vi "DHE_Interlocks.vi"(8 "remaining":string, 9 "field":string, 10 "parent":string, 11 "DHE_ImgState":T1(ring)) -> (2 "interlock closed":bool)   [LabVIEW 2016]
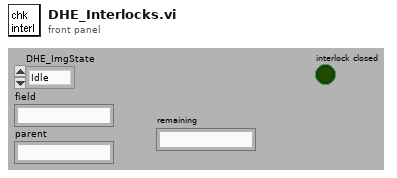
[diagram p1: front panel]
types:
  T1 = enum16{"Idle", "Exposing", "Paused", "AbortExp", "Reading", "AbortRead", "FinishedReading", "Resetting", "Reducing", "Initializing"}
  T2 = enum16{"add", "delete", "find", "clear all", "getall", "all"}
  T3 = cluster{"state":string, "rules":cluster{"command":string, "action":string}[]}[]
  T4 = cluster{"state":string, "rules":cluster{"command":string, "action":string}[]}
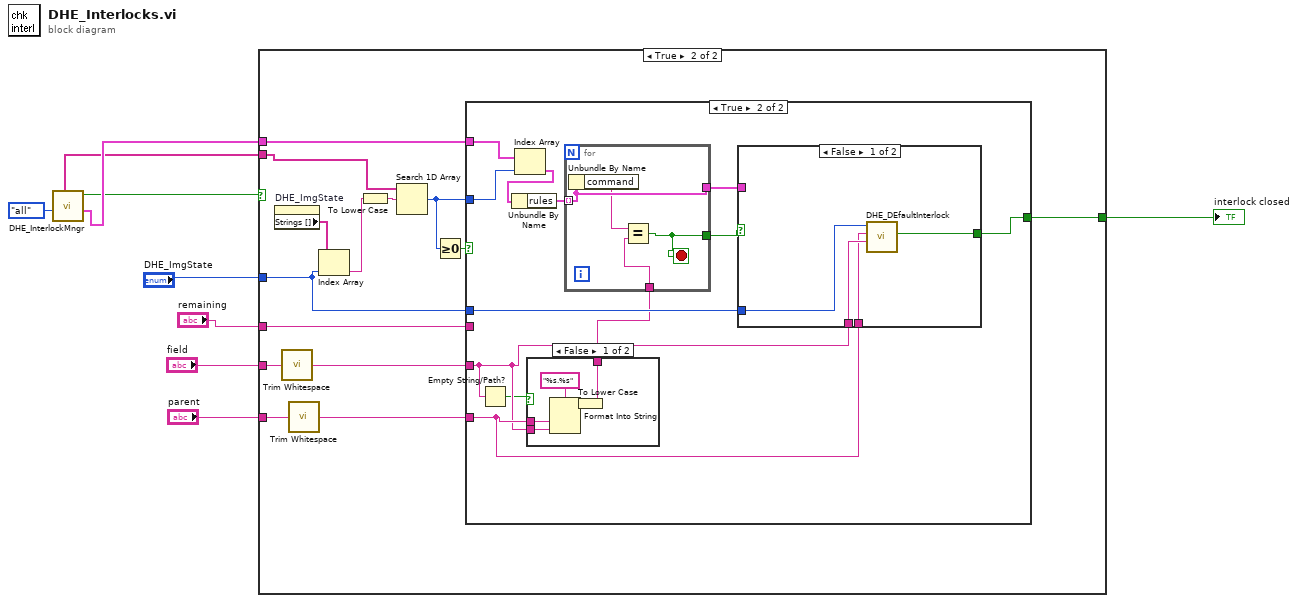
[diagram p0: block diagram]
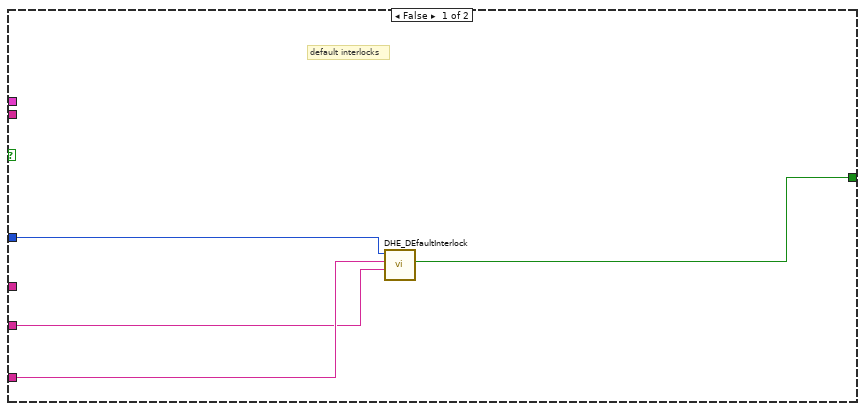
[diagram p2: hidden frame]
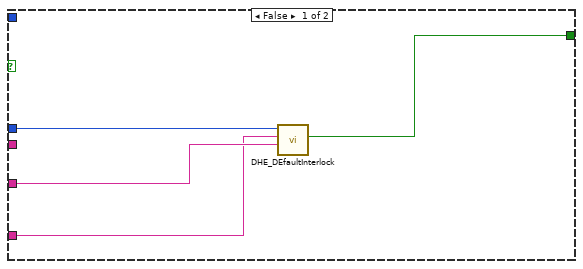
[diagram p3: hidden frame]
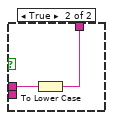
[diagram p4: hidden frame]
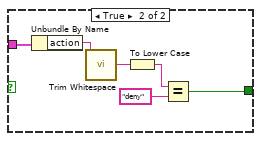
[diagram p5: hidden frame]
diagram:
  n1 = call "DHE_InterlockMngr.vi"("Enum"=T2."all") -> ("interlocks"=w4:T3, "defined?"=w2:bool, "states"=w3:string[])  [unwired: 3 in, 5 out]
  n2 = case shown="True" w2 {
    tunnel: "DHE_ImgState" -> [w13 w23]
    tunnel: "field" -> [w11 w16]
    tunnel: "parent" -> [w12 w22]
    tunnel: [w10 w21] -> w6
    tunnel: w4 -> [_ w18]
    tunnel: w3 -> [_ w19]
    tunnel: "remaining" -> [_ w14]
    frame False {
      # "default interlocks"
      n3 = call "DHE_DEfaultInterlock.vi"("field"=w11, "parent"=w12, "DHE_ImgState"=w13) -> ("interlock"=w10:bool)  [unwired: 8 out]
    }
    frame True {
      n4 = property on="DHE_ImgState" class="Enum (strict)"() -> ("Strings []"=w27:string[])  [unwired: 2 in, 2 out]
      n5 = call <vilib>:"Trim Whitespace.vi"("string"=w16) -> ("trimmed string"=w15:string)  [unwired: 1 in]
      n6 = call <vilib>:"Trim Whitespace.vi"("string"=w22) -> ("trimmed string"=w17:string)  [unwired: 1 in]
      n7 = Index Array(array=w27, index=w23) -> (element=w26:string)
      n8 = To Lower Case(string=w26) -> (all lower case string=w25:string)
      n9 = Search 1D Array(1D array=w19, element=w25) -> (index of element=w20:i32)  [unwired: 1 out]
      n10 = Greater Or Equal To 0?(x=w20) -> (x >= 0?=w24:bool)
      n11 = case shown="True" w24 {
        tunnel: w23 -> [w31 w42]
        tunnel: w15 -> [w30 w34]
        tunnel: w17 -> [w29 w41]
        tunnel: [w28 w40] -> w21
        tunnel: w20 -> [_ w38]
        tunnel: w18 -> [_ w39]
        tunnel: w14 -> [_ _]
        frame False {
          n12 = call "DHE_DEfaultInterlock.vi"("field"=w30, "parent"=w29, "DHE_ImgState"=w31) -> ("interlock"=w28:bool)  [unwired: 8 out]
        }
        frame True {
          n13 = Empty String/Path?(string/path=w34) -> (empty?=w33:bool)
          n14 = Index Array(array=w39, index=w38) -> (element=w37:T4)
          n15 = Unbundle By Name(w37) -> ("rules"=w36:cluster{"command":string, "action":string}[])
          n16 = case shown="False" w33 {
            tunnel: w34 -> [w46 _]
            tunnel: w41 -> [w45 w50]
            tunnel: [w44 w49] -> w32
            frame False {
              n17 = Format Into String(format string="%s.%s", w45, w46) -> (resulting string=w47:string)  [unwired: 2 in, 1 out]
              n18 = To Lower Case(string=w47) -> (all lower case string=w44:string)
            }
            frame True {
              n19 = To Lower Case(string=w50) -> (all lower case string=w49:string)
            }
          }
          n20 = for {
            tunnel: w32 -> [w62]
            tunnel: [w61] -> w43
            tunnel: w36 -> [w64] mode=indexing
            tunnel: [w64] -> w35
            stop <- w61 stop-if-true
            n21 = Unbundle By Name(w64) -> ("command"=w63:string)
            n22 = Equal?(x=w63, y=w62) -> (x = y?=w61:bool)
          }
          n23 = case shown="False" w43 {
            tunnel: w42 -> [w54 _]
            tunnel: w34 -> [w53 _]
            tunnel: w41 -> [w52 _]
            tunnel: [w51 w57] -> w40
            tunnel: w35 -> [_ w55]
            frame False {
              n24 = call "DHE_DEfaultInterlock.vi"("field"=w53, "parent"=w52, "DHE_ImgState"=w54) -> ("interlock"=w51:bool)  [unwired: 8 out]
            }
            frame True {
              n25 = Unbundle By Name(w55) -> ("action"=w56:string)
              n26 = call <vilib>:"Trim Whitespace.vi"("string"=w56) -> ("trimmed string"=w60:string)  [unwired: 1 in]
              n27 = To Lower Case(string=w60) -> (all lower case string=w59:string)
              n28 = Equal?(x=w59, y="deny") -> (x = y?=w57:bool)
            }
          }
        }
      }
    }
  }
  "interlock closed" <- w6
